vi "DriveAutoTarget.vi"(2 "Parameter String":string="near") -> (0 "Error Out":errorcluster, 1 "Increment":bool)   [LabVIEW 2020]
doc: "The swerve drive base will translate in the field-centric X direction until it reaches the CHARGING STATION. Then it will move up the ramp and balance using the pitch feedback from the IMU.\n\nParameters:\n1. \"near\" or \"far\" to indicate which side the robot is coming from in relation to the driver station"
uses:
  SafeParser_String.vi
  GlobalAutonomous.vi
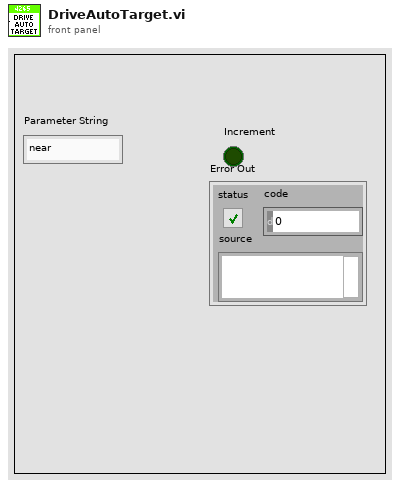
[diagram p1: front panel]
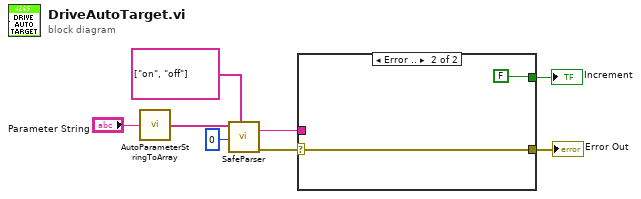
[diagram p0: block diagram]
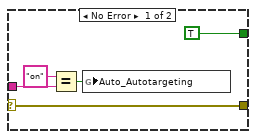
[diagram p2: hidden frame]
diagram:
  n1 = call "AutoParameterStringToArray.vi"("Parameter String"="Parameter String") -> ("Parsed Parameters"=w6:string[])
  n2 = call-poly "SafeParser.vi"("Allowed Values"=string[] ["on", "off"], "Array Index"=0 ("Parameter Index"), "String Array"=w6) -> ("Error Out"=w1:errorcluster, "Typecast Value"=w5:string)  [unwired: 7 in]
  n3 = case shown="Error .." w1 {
    selector: w1 -> [w13 w15]
    tunnel: [TRUE FALSE] -> w3
    tunnel: [w13 w15] -> w8
    tunnel: w5 -> [w11 _]
    frame No Error {
      n4 = Equal?(x="on", y=w11) -> (x = y?=w10:bool)
      n5 = global write "GlobalAutonomous.vi" "Auto_Autotargeting"(w10) -> ()
    }
    frame Error {
    }
  }
  "Increment" <- w3
  "Error Out" <- w8
